vi "LoadExcelToDB.vi"() -> ()   [LabVIEW 2012]
uses:
  <vilib>/addons/database/Connection.llb/DB Tools Open Connec (Path).vi
  <vilib>/addons/database/Connection.llb/Conn Execute.vi
  <vilib>/addons/database/Recordset.llb/Rec Fetch Integer Data (R).vi
  <vilib>/addons/database/Recordset.llb/Rec Destroy - Connection.vi
  <vilib>/addons/database/NI_Database_API.lvlib
panel:
  out "appended path":path
  out "error out":errorcluster
  in  "Cluster":T1
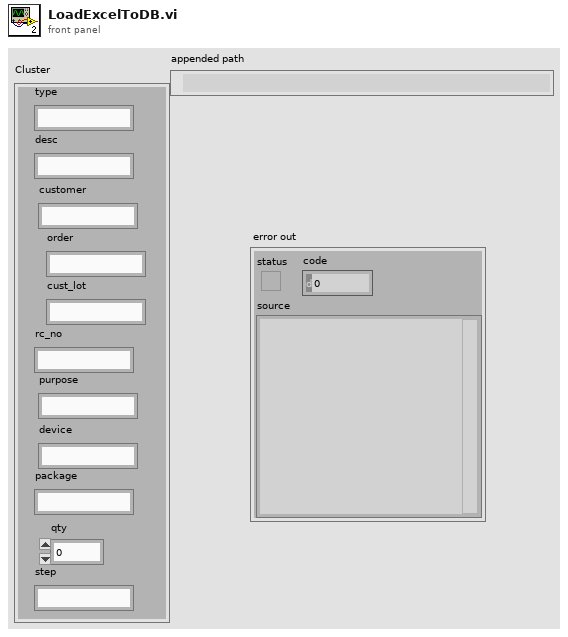
[diagram p1: front panel]
types:
  T1 = cluster{"type":string, "desc":string, "customer":string, "order":string, "cust_lot":string, "rc_no":string, "purpose":string, "device":string, "package":string, "qty":dbl, "step":string}
  T2 = typedef "NI_Database_API.lvlib/Conn ObjectReference.ctl" = refnum<k1>
  T3 = typedef "NI_Database_API.lvlib/Rec ObjectReference.ctl" = refnum<k1>
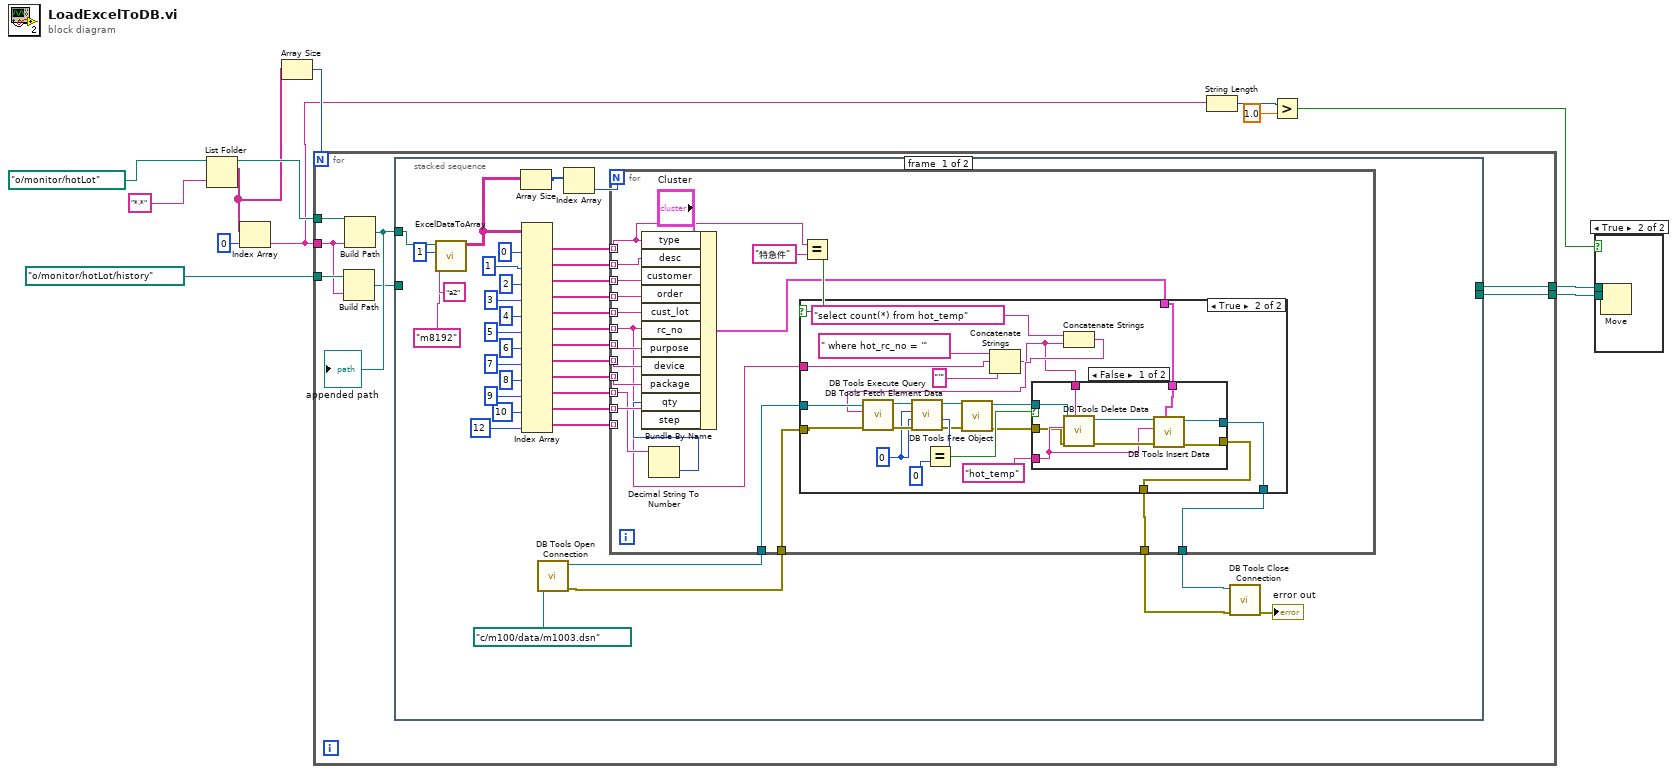
[diagram p0: block diagram]
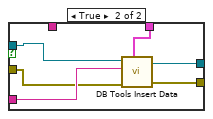
[diagram p4: hidden frame]
diagram:
  n1 = List Folder(path=path "o:/monitor/hotLot", pattern="*.*") -> (path out=w10:path, filenames=w9:string[])  [unwired: 2 in, 2 out]
  n2 = Index Array(array=w9, index=0) -> (element=w4:string)
  n3 = Array Size(array=w9) -> (size(s)=w12:i32)
  n4 = for {
    N: w12 -> [_]
    tunnel: w4 -> [w17]
    tunnel: w10 -> [w20]
    tunnel: path "o:/monitor/hotLot/history" ("base path") -> [w18]
    tunnel: [w15] -> w6
    tunnel: [w14] -> w5
    n5 = Build Path(base path=w18, name or relative path=w17) -> (appended path=w16:path)
    n6 = Build Path(base path=w20, name or relative path=w17) -> (appended path=w19:path)
    "appended path" <- w19
    n7 = stacked-sequence {
      tunnel: w19 -> [w23 w118]
      tunnel: w16 -> [_ w117]
      tunnel: [_ w118] -> w15
      tunnel: [_ w117] -> w14
      frame #0 {
        n8 = call "ExcelDataToArray.vi"("end cell"="m8192", "start cell"="a2", "sheet#"=1, "path"=w23) -> ("data"=w49:string[][])  [unwired: 6 in, 1 out]
        n9 = Array Size(array=w49) -> (size(s)=w53:i32[])
        n10 = Index Array(array=w49, index (col) #1=0 ("disabled index (col)"), index (col) #2=1 ("index (col)"), index (col) #3=2 ("index (col)"), index (col) #4=3 ("index (col)"), index (col) #5=4 ("index (col)"), index (col) #6=5 ("index (col)"), index (col) #7=6 ("index (col)"), index (col) #8=7 ("index (col)"), index (col) #9=8 ("index (col)"), index (col) #10=9 ("index (col)"), index (col) #11=10 ("index (col)"), index (col) #12=12 ("index (col)")) -> (element #1=w38:string[], element #2=w37:string[], element #3=w36:string[], element #4=w35:string[], element #5=w34:string[], element #6=w33:string[], element #7=w32:string[], element #8=w31:string[], element #9=w30:string[], element #10=w29:string[], element #11=w28:string[], element #12=w21:string[])  [unwired: 12 in]
        n11 = call-poly <vilib>:"DB Tools Open Connection.vi"("connection information"=path "c:/m100/data/m1003.dsn") -> ("error out"=w26:errorcluster, "connection reference"=w27:T2)  [unwired: 7 in]
        n12 = Index Array(array=w53) -> (element=w52:i32)  [unwired: 1 in]
        n13 = for {
          N: w52 -> [_]
          tunnel: w38 -> [w67] mode=indexing
          tunnel: w37 -> [w75] mode=indexing
          tunnel: w36 -> [w74] mode=indexing
          tunnel: w35 -> [w73] mode=indexing
          tunnel: w34 -> [w72] mode=indexing
          tunnel: w33 -> [w60] mode=indexing
          tunnel: w32 -> [w68] mode=indexing
          tunnel: w31 -> [w69] mode=indexing
          tunnel: w30 -> [w70] mode=indexing
          tunnel: w29 -> [w62] mode=indexing
          tunnel: w28 -> [w71] mode=indexing
          tunnel: w27 -> [w64]
          tunnel: w26 -> [w63]
          tunnel: [w58] -> w25
          tunnel: [w59] -> w24
          tunnel: w21 -> [_] mode=indexing
          n14 = Decimal String To Number(string=w62) -> (number=w61:i32)  [unwired: 2 in, 1 out]
          n15 = Bundle By Name(cluster="Cluster", "type"=w67, "desc"=w75, "customer"=w74, "order"=w73, "cust_lot"=w72, "rc_no"=w60, "purpose"=w68, "device"=w69, "package"=w70, "qty"=w61, "step"=w71) -> (w65:T1)
          n16 = Equal?(x=w67, y="特急件") -> (x = y?=w66:bool)
          n17 = case shown="True" w66 {
            tunnel: w65 -> [_ w101]
            tunnel: w64 -> [w78 w100]
            tunnel: w63 -> [w79 w96]
            tunnel: w60 -> [_ w98]
            tunnel: [w79 w86] -> w59
            tunnel: [w78 w85] -> w58
            frame False {
            }
            frame True {
              w80 = 0
              n18 = Concatenate Strings(" where hot_rc_no = '" ("string"), w98, "'" ("string")) -> (w87:string)
              n19 = Concatenate Strings("select count(*) from hot_temp" ("string"), w87) -> (w88:string)
              n20 = call-poly <vilib>:"DB Tools Execute Query.vi"("error in (no error)"=w96, "SQL query"=w88, "connection reference"=w100) -> ("error out"=w95:errorcluster, "recordset reference"=w94:T3)  [unwired: 5 in]
              n21 = call-poly <vilib>:"DB Tools Fetch Element Data.vi"("error in (no error)"=w95, "type"=w80, "column index"=w80, "recordset reference"=w94) -> ("error out"=w84:errorcluster, "data"=w93:i32, "recordset reference out"=w83:T3)  [unwired: 3 in]
              n22 = Equal?(x=w93, y=0) -> (x = y?=w91:bool)
              n23 = call-poly <vilib>:"DB Tools Free Object.vi"("error in (no error)"=w84, "recordset reference"=w83) -> ("error out"=w81:errorcluster, "connection reference"=w82:T2)  [unwired: 8 in]
              n24 = case shown="False" w91 {
                tunnel: w101 -> [w106 w116]
                tunnel: [w105 w115] -> w85
                tunnel: [w104 w114] -> w86
                tunnel: "hot_temp" ("table") -> [w107 w113]
                tunnel: w87 -> [w110 _]
                tunnel: w82 -> [w103 w112]
                tunnel: w81 -> [w102 w111]
                frame False {
                  n25 = call <vilib>:"DB Tools Delete Data.vi"("condition"=w110, "error in (no error)"=w102, "table"=w107, "connection reference"=w103) -> ("error out"=w109:errorcluster, "connection reference out"=w108:T2)  [unwired: 6 in]
                  n26 = call <vilib>:"DB Tools Insert Data.vi"("data"=w106, "error in (no error)"=w109, "table"=w107, "connection reference"=w108) -> ("error out"=w104:errorcluster, "connection reference out"=w105:T2)  [unwired: 6 in]
                }
                frame True {
                  n27 = call <vilib>:"DB Tools Insert Data.vi"("data"=w116, "error in (no error)"=w111, "table"=w113, "connection reference"=w112) -> ("error out"=w114:errorcluster, "connection reference out"=w115:T2)  [unwired: 6 in]
                }
              }
            }
          }
        }
        n28 = call <vilib>:"DB Tools Close Connection.vi"("error in (no error)"=w24, "connection reference"=w25) -> ("error out"=→"error out":errorcluster)  [unwired: 5 in]
      }
      frame #1 {
      }
    }
  }
  n29 = String Length(string=w4) -> (length=w2:i32)
  n30 = Greater?(x=w2, y=1.0) -> (0:w1:bool)
  n31 = case shown="True" w1 {
    tunnel: w6 -> [_ w120]
    tunnel: w5 -> [_ w119]
    frame False {
    }
    frame True {
      n32 = Move(source path=w120, 10:w119) -> ()  [unwired: 3 in, 3 out]
    }
  }
